vi "loglog_linearfit.vi"(6 "Current":dbl[](array[numeric]), 9 "Voltage":dbl[](array[numeric]), 10 "index":i32=5, 11 "length":i32=50) -> (0 "Best Linear Fit":dbl[](array[numeric]), 1 "error":i32, 2 "V indexed":dbl[](array[numeric]), 3 "Ic":dbl, 5 "I indexed":dbl[](array[numeric]))   [LabVIEW 2022 SP3]
uses:
  <vilib>/Analysis/NI_AALPro.lvlib
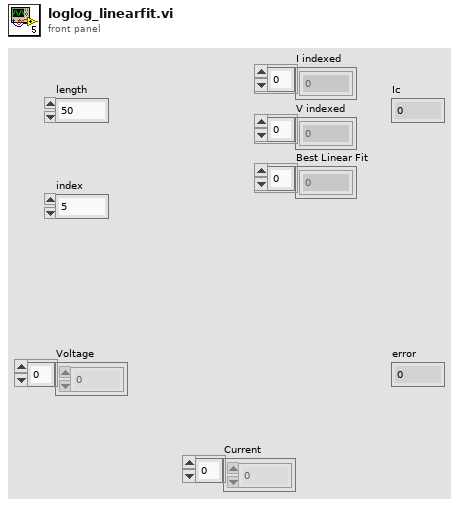
[diagram p1: front panel]
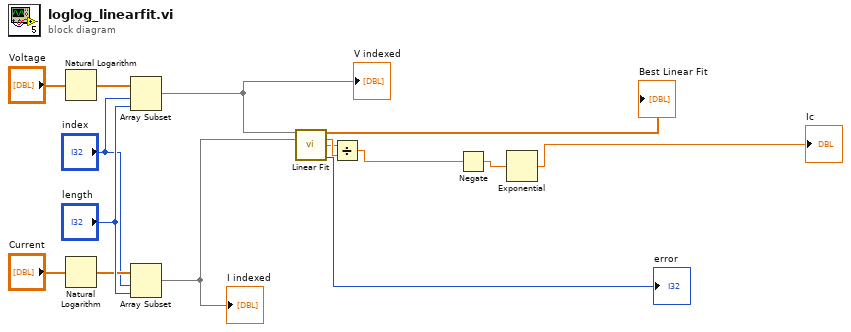
[diagram p0: block diagram]
diagram:
  n1 = Natural Logarithm(1:"Voltage") -> (0:w12:dbl[])
  n2 = Natural Logarithm(1:"Current") -> (0:w13:dbl[])
  n3 = Array Subset(array=w12, index="index", length="length") -> (w3:dbl[])
  "V indexed" <- w3
  n4 = Array Subset(array=w13, index="index", length="length") -> (w2:dbl[])
  "I indexed" <- w2
  n5 = call <vilib>:"Linear Fit.vi"("Y"=w3, "X"=w2) -> ("Best Linear Fit"=→"Best Linear Fit":dbl[], "slope"=w5:dbl, "intercept"=w4:dbl, "error"=→"error":i32)  [unwired: 9 in, 1 out]
  n6 = Divide(x=w4, y=w5) -> (x/y=w6:dbl)
  n7 = Negate(x=w6) -> (-x=w7:dbl)
  n8 = Exponential(1:w7) -> (0:→"Ic":dbl)
